vi "GetSelectionList.vi"(8 "error in (no error)":errorcluster caption="错误输入（无错误）", 11 "XYPlot 输入":refnum<class "TrendPlot.lvclass">) -> (0 "error out":errorcluster caption="错误输出", 3 "XYPlot 输出":refnum<class "TrendPlot.lvclass">)   [LabVIEW 2018, in "DataDisplay.lvlib" / "TrendPlot.lvclass"]
uses:
  TrendPlot.lvclass
  TrendPlot.lvclass/TrendPlot.ctl
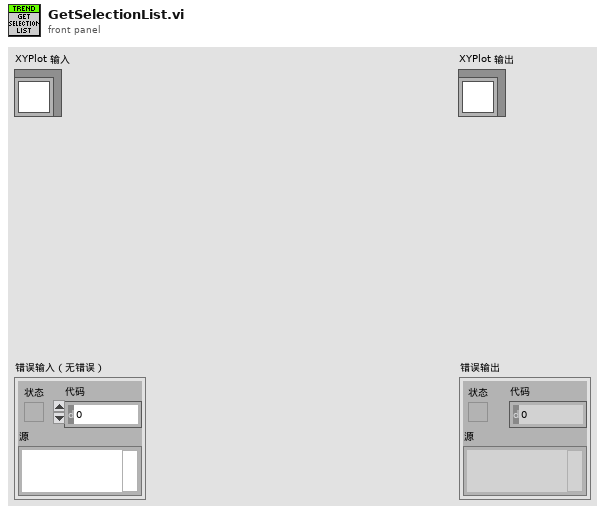
[diagram p1: front panel]
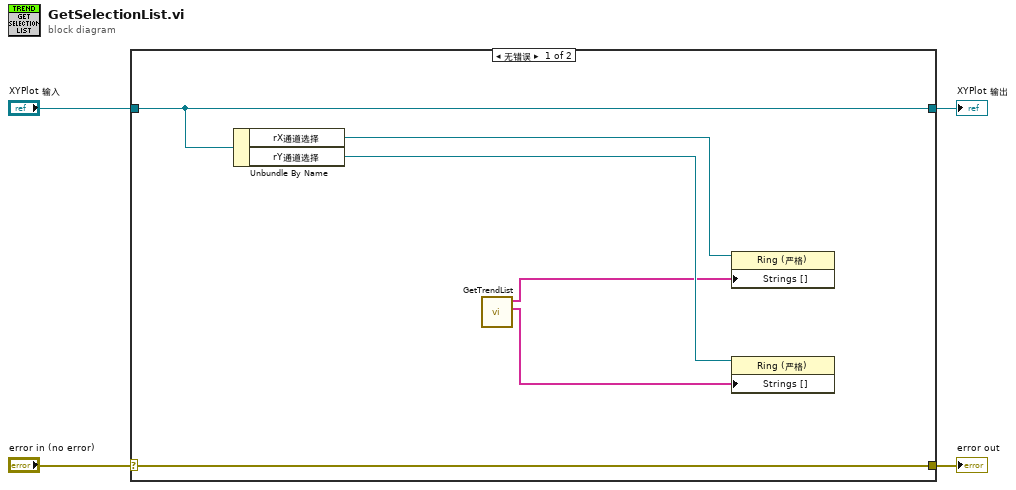
[diagram p0: block diagram]
diagram:
  n1 = case shown="无错误" "error in (no error)" {
    selector: "error in (no error)" -> [w10 w12]
    tunnel: [w10 w12] -> w3
    tunnel: [w9 w11] -> w1
    tunnel: "XYPlot 输入" -> [w9 w11]
    frame No Error {
      n2 = Unbundle By Name(w9) -> ("rX通道选择"=w8:refnum<vi>, "rY通道选择"=w7:refnum<vi>)
      n3 = call "GetTrendList.vi"() -> ("Y列表"=w5:string[], "X列表"=w6:string[])  [unwired: 10 in]
      n4 = property class="Ring (严格)"(reference=w8, "Strings []"=w6) -> ()  [unwired: 1 in, 2 out]
      n5 = property class="Ring (严格)"(reference=w7, "Strings []"=w5) -> ()  [unwired: 1 in, 2 out]
    }
    frame Error {
    }
  }
  "error out" <- w3
  "XYPlot 输出" <- w1
